vi "Array 1.vi"() -> (11 "Table Control 1":string[][](table))   [LabVIEW 2017]
uses:
  <vilib>/Utility/file.llb/Write Delimited Spreadsheet (string).vi
panel:
  in  "Direktori File":path
  in  "Stop 2":bool
  out "Table Control 2":string[][](table)
  out "Waveform Chart 2":cluster{dbl, dbl, dbl, dbl}(graph)
  out "Waveform Chart":cluster{dbl, dbl, dbl, dbl}(graph)
  in  "Stop 1":bool
  out "output array":dbl[](array[numeric])
  out "element":dbl
  in  "Array":dbl[](array[numeric])
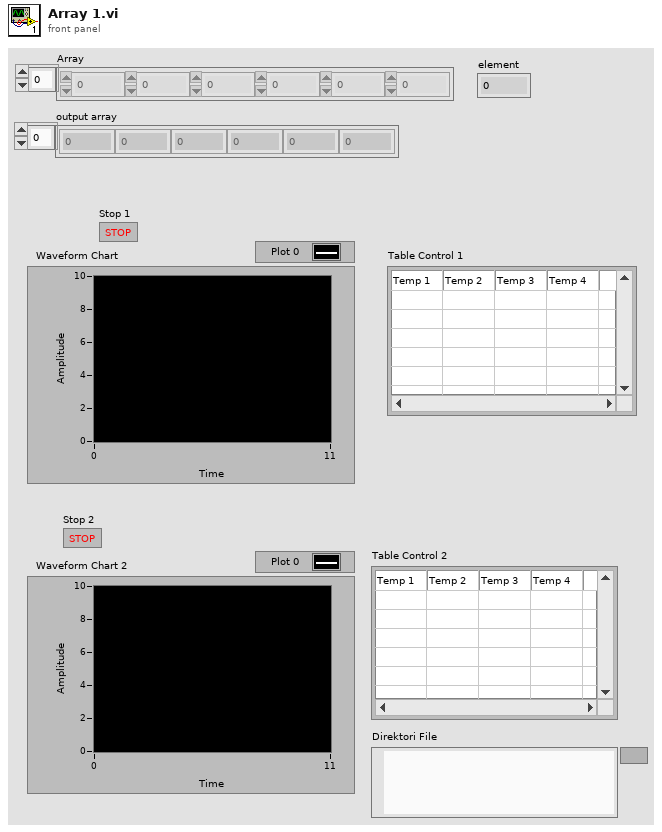
[diagram p1: front panel]
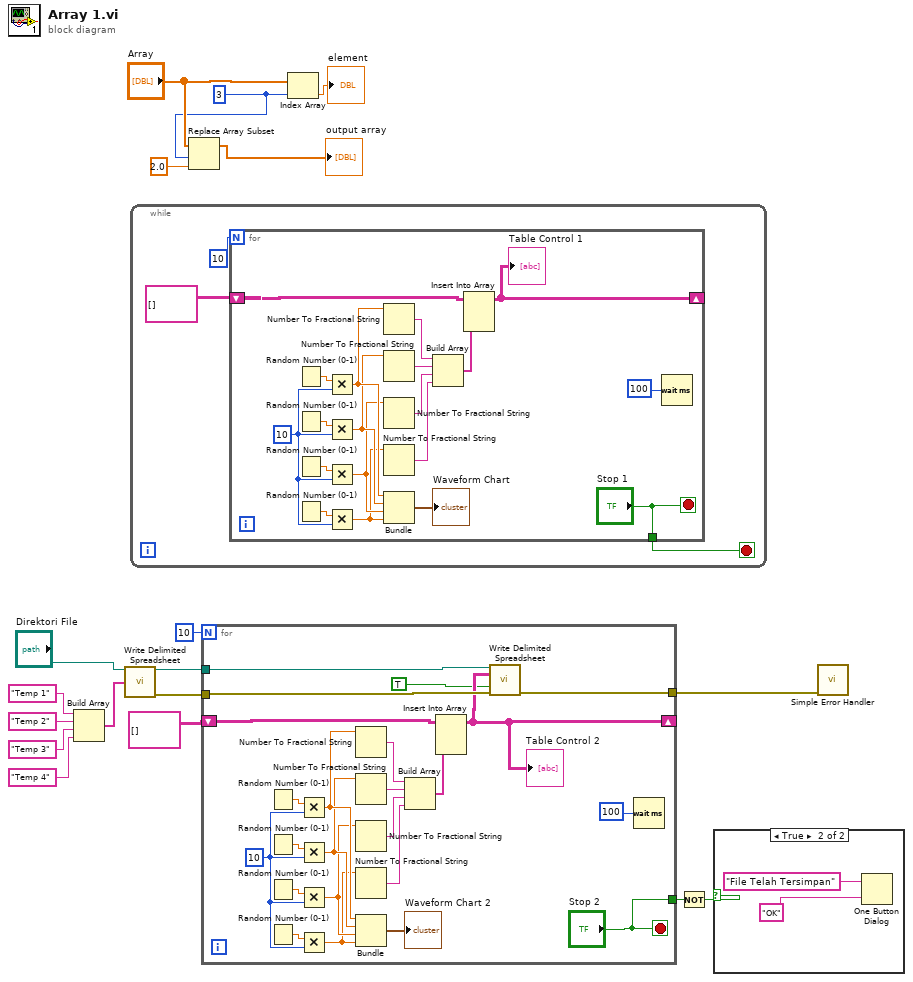
[diagram p0: block diagram]
diagram:
  w15 = 3
  n1 = Build Array("Temp 1", "Temp 2", "Temp 3", "Temp 4") -> (w12:string[])
  n2 = call-poly <vilib>:"Write Delimited Spreadsheet.vi"("file path (dialog if empty)"="Direktori File", "1D data"=w12) -> ("new file path (Not A Path if cancelled)"=w5:path, "error out"=w6:errorcluster)  [unwired: 12 in]
  n3 = while {
    stop <- w19 stop-if-true
    n4 = for {
      N: 10 -> [_]
      shift-right: [w33] -> _
      shift-left: string[][] [] -> [w39]
      tunnel: ["Stop 1"] -> w19
      stop <- "Stop 1" stop-if-true
      w27 = 10
      n5 = Random Number (0-1)() -> (number: 0 to 1=w31:dbl)
      n6 = Random Number (0-1)() -> (number: 0 to 1=w30:dbl)
      n7 = Random Number (0-1)() -> (number: 0 to 1=w29:dbl)
      n8 = Random Number (0-1)() -> (number: 0 to 1=w28:dbl)
      n9 = Multiply(x=w31, y=w27) -> (x*y=w26:dbl)
      n10 = Multiply(x=w30, y=w27) -> (x*y=w25:dbl)
      n11 = Multiply(x=w29, y=w27) -> (x*y=w24:dbl)
      n12 = Multiply(x=w28, y=w27) -> (x*y=w23:dbl)
      n13 = Number To Fractional String(number=w26) -> (F-format string=w38:string)  [unwired: 3 in]
      n14 = Number To Fractional String(number=w25) -> (F-format string=w36:string)  [unwired: 3 in]
      n15 = Number To Fractional String(number=w24) -> (F-format string=w35:string)  [unwired: 3 in]
      n16 = Number To Fractional String(number=w23) -> (F-format string=w34:string)  [unwired: 3 in]
      n17 = Bundle(w26, w25, w24, w23) -> (→"Waveform Chart":cluster{dbl, dbl, dbl, dbl})  [unwired: 1 in]
      n18 = Build Array(w38, w36, w35, w34) -> (w37:string[])
      n19 = Insert Into Array(array=w39, new element=w37) -> (w33:string[][])  [unwired: 2 in]
      "Table Control 1" <- w33
      n20 = Wait (ms)(milliseconds to wait=100) -> ()  [unwired: 1 out]
    }
  }
  n21 = Replace Array Subset(array="Array", new element=2.0 ("new element/subarray"), index=w15) -> (→"output array":dbl[])
  n22 = for {
    N: 10 -> [_]
    shift-right: [w44] -> _
    shift-left: string[][] [] -> [w62]
    tunnel: w5 -> [w46]
    tunnel: w6 -> [w45]
    tunnel: [w41] -> w3
    tunnel: ["Stop 2"] -> w2
    stop <- "Stop 2" stop-if-true
    w52 = 10
    n23 = Random Number (0-1)() -> (number: 0 to 1=w56:dbl)
    n24 = Random Number (0-1)() -> (number: 0 to 1=w55:dbl)
    n25 = Random Number (0-1)() -> (number: 0 to 1=w54:dbl)
    n26 = Random Number (0-1)() -> (number: 0 to 1=w53:dbl)
    n27 = Multiply(x=w56, y=w52) -> (x*y=w51:dbl)
    n28 = Multiply(x=w55, y=w52) -> (x*y=w50:dbl)
    n29 = Multiply(x=w54, y=w52) -> (x*y=w49:dbl)
    n30 = Multiply(x=w53, y=w52) -> (x*y=w48:dbl)
    n31 = Number To Fractional String(number=w51) -> (F-format string=w61:string)  [unwired: 3 in]
    n32 = Number To Fractional String(number=w50) -> (F-format string=w59:string)  [unwired: 3 in]
    n33 = Number To Fractional String(number=w49) -> (F-format string=w58:string)  [unwired: 3 in]
    n34 = Number To Fractional String(number=w48) -> (F-format string=w57:string)  [unwired: 3 in]
    n35 = Bundle(w51, w50, w49, w48) -> (→"Waveform Chart 2":cluster{dbl, dbl, dbl, dbl})  [unwired: 1 in]
    n36 = Build Array(w61, w59, w58, w57) -> (w60:string[])
    n37 = Insert Into Array(array=w62, new element=w60) -> (w44:string[][])  [unwired: 2 in]
    "Table Control 2" <- w44
    n38 = call-poly <vilib>:"Write Delimited Spreadsheet.vi"("file path (dialog if empty)"=w46, "2D data"=w44, "append to file? (new file:F)"=TRUE, "error in (no error)"=w45) -> ("error out"=w41:errorcluster)  [unwired: 10 in, 1 out]
    n39 = Wait (ms)(milliseconds to wait=100) -> ()  [unwired: 1 out]
  }
  n40 = Index Array(array="Array", index=w15) -> (element=→"element":dbl)
  n41 = Not(x=w2) -> (.not. x?=w1:bool)
  n42 = case shown="True" w1 {
    frame False {
    }
    frame True {
      n43 = One Button Dialog(message="File Telah Tersimpan", button name ("OK")="OK") -> ()  [unwired: 1 out]
    }
  }
  n44 = call <vilib>:"Simple Error Handler.vi"("error in (no error)"=w3) -> ()  [unwired: 4 in, 5 out]
